vi "laser_comms_server.vi"() -> ()   [LabVIEW 2023]
panel:
  out "Recieved Message":string
  out "Sent Message":string
  in  "Stop Button":bool
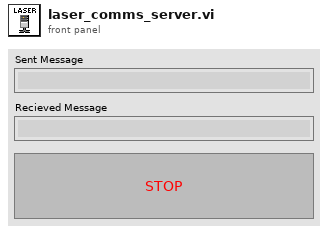
[diagram p1: front panel]
types:
  T1 = enum16{"Standard", "Buffered", "CRLF", "Immediate"}
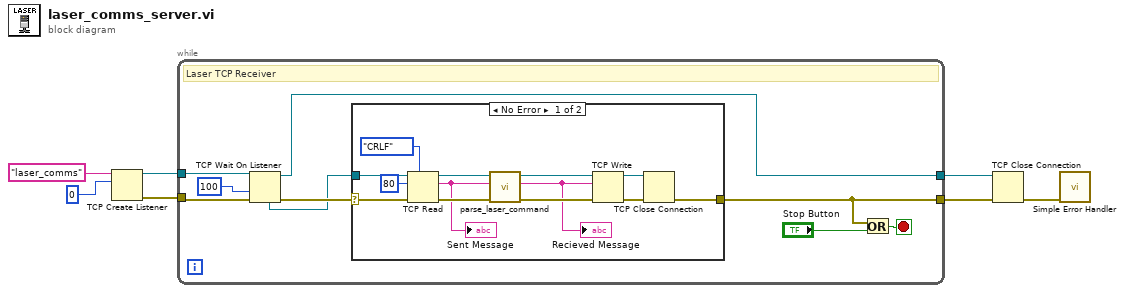
[diagram p0: block diagram]
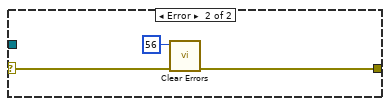
[diagram p2: hidden frame]
diagram:
  n1 = TCP Create Listener(10:u16 0 ("remote port or service name"), 11:"laser_comms" ("service name")) -> (0:w6:errorcluster, 3:w7:refnum<k5>)  [unwired: 3 in, 1 out]
  n2 = while {
    tunnel: w7 -> [w14]
    tunnel: w6 -> [w13]
    tunnel: [w9] -> w2
    tunnel: [w8] -> w3
    stop <- w15 stop-if-true
    # "Laser TCP Receiver"
    n3 = TCP Wait On Listener(8:w13, 9:100 ("timeout ms (wait forever: -1)"), 11:w14) -> (0:w12:errorcluster, 3:w8:refnum<k5>, 4:w11:refnum<k5>)  [unwired: 1 in, 2 out]
    n4 = case shown="No Error" w12 {
      selector: w12 -> [w27 w30]
      tunnel: w11 -> [w24 _]
      tunnel: [w21 w29] -> w9
      frame No Error {
        n5 = TCP Read(connection ID=w24, bytes to read=80, error in (no error)=w27, 7:T1."CRLF" ("mode (standard)")) -> (connection ID out=w25:refnum<k5>, data out=w18:string, error out=w26:errorcluster)  [unwired: 1 in]
        "Sent Message" <- w18
        n6 = call "parse_laser_command.vi"("Input String"=w18) -> ("Output String"=w17:string)  [unwired: 10 in]
        "Recieved Message" <- w17
        n7 = TCP Write(connection ID=w25, data in=w17, error in (no error)=w26) -> (connection ID out=w23:refnum<k5>, error out=w22:errorcluster)  [unwired: 1 in, 1 out]
        n8 = TCP Close Connection(connection ID=w23, error in (no error)=w22) -> (error out=w21:errorcluster)  [unwired: 1 in, 1 out]
      }
      frame Error {
        n9 = call <vilib>:"Clear Errors.vi"("error in (no error)"=w30, "specific error code to clear (0: all)"=56) -> ("error out"=w29:errorcluster)  [unwired: 4 in, 1 out]
      }
    }
    n10 = Or(x=w9, y="Stop Button") -> (x .or. y?=w15:bool)
  }
  n11 = TCP Close Connection(connection ID=w3, error in (no error)=w2) -> (error out=w1:errorcluster)  [unwired: 1 in, 1 out]
  n12 = call <vilib>:"Simple Error Handler.vi"("error in (no error)"=w1) -> ()  [unwired: 4 in, 5 out]
